vi "ChannelEnabled.vi"(10 "Enabled Channel 2":bool, 11 "Enabled Channel 1":bool) -> (2 "Channels":string[](array[string]))   [LabVIEW 2020]
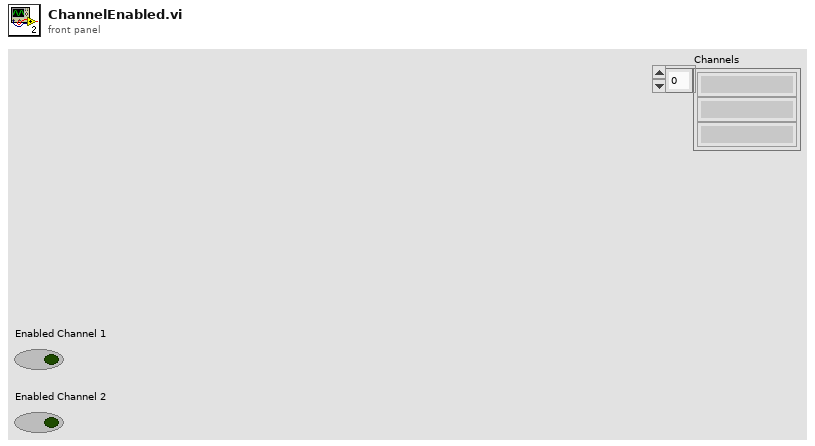
[diagram p1: front panel]
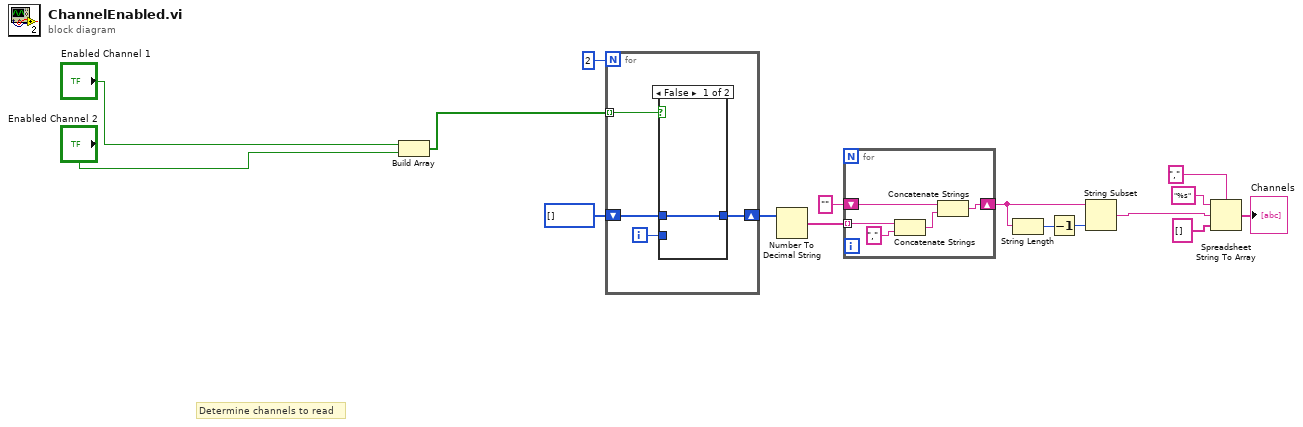
[diagram p0: block diagram]
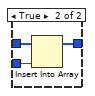
[diagram p2: hidden frame]
diagram:
  # "Determine channels to read"
  n1 = Build Array("Enabled Channel 1", "Enabled Channel 2") -> (w1:bool[])
  n2 = for {
    N: 2 -> [_]
    shift-right: [w18] -> w7
    shift-left: i32[] [] -> [w19]
    tunnel: w1 -> [w17] mode=indexing
    i -> [w20]
    n3 = case shown="False" w17 {
      tunnel: w20 -> [_ w24]
      tunnel: w19 -> [w21 w23]
      tunnel: [w21 w22] -> w18
      frame False {
      }
      frame True {
        n4 = Insert Into Array(array=w23, new element=w24) -> (w22:i32[])  [unwired: 1 in]
      }
    }
  }
  n5 = Number To Decimal String(number=w7) -> (decimal integer string=w6:string[])  [unwired: 1 in]
  n6 = for {
    tunnel: w6 -> [w28] mode=indexing
    shift-right: [w27] -> w8
    shift-left: "" -> [w26]
    n7 = Concatenate Strings(w28, "," ("string")) -> (w25:string)
    n8 = Concatenate Strings(w26, w25) -> (w27:string)
  }
  n9 = String Length(string=w8) -> (length=w10:i32)
  n10 = Decrement(x=w10) -> (x-1=w9:i32)
  n11 = String Subset(string=w8, length (rest)=w9) -> (substring=w5:string)  [unwired: 1 in]
  n12 = Spreadsheet String To Array(delimiter (Tab)=",", format string="%s", spreadsheet string=w5, array type (2D Dbl)=string[] []) -> (array=→"Channels":string[])
